vi "Status Acquisition Ex.vi"(0 "status":i32, 1 "indexOfLastCompletedFrame":i32, 2 "error in (no error)":errorcluster) -> (3 "status out":i32, 4 "indexOfLastCompletedFrame out":i32, 5 "function return":i32, 6 "error out":errorcluster)   [LabVIEW 2020, in "ThorConfocal.lvlib"]
doc: "long StatusAcquisitionEx(long &status, long &indexOfLastCompletedFrame);"
uses:
  ThorConfocal.lvlib
  ThorConfocal.dll
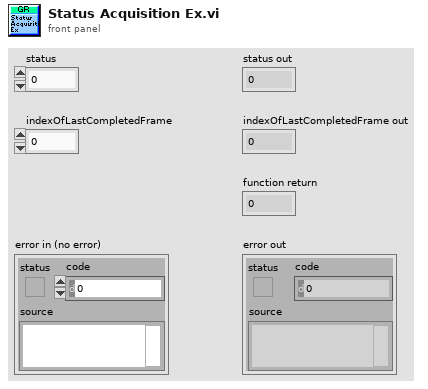
[diagram p1: front panel]
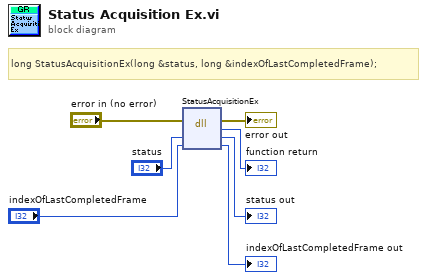
[diagram p0: block diagram]
diagram:
  # "long StatusAcquisitionEx(long &status, long &indexOfLastCompletedFrame);"
  n1 = dll-call lib="D:/software/TweezerTron/ThorConfocal.dll" fn="StatusAcquisitionEx"(error in="error in (no error)", "status"="status", "indexOfLastCompletedFrame"="indexOfLastCompletedFrame") -> (error out=→"error out":errorcluster, "return type"=→"function return":i32, "status"=→"status out":i32, "indexOfLastCompletedFrame"=→"indexOfLastCompletedFrame out":i32)  [unwired: 2 in, 1 out]
